vi "splitt argument.vi"(1 "formula":string) -> (0 "Array":string[](array[string]))   [LabVIEW 2011]
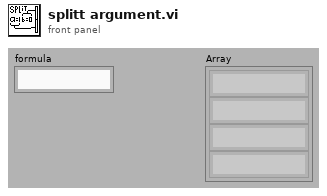
[diagram p1: front panel]
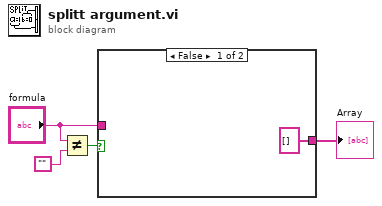
[diagram p0: block diagram]
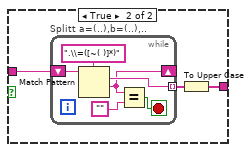
[diagram p2: hidden frame]
diagram:
  n1 = Not Equal?(x="formula", y="") -> (x != y?=w3:bool)
  n2 = case shown="False" w3 {
    tunnel: "formula" -> [_ w8]
    tunnel: [string[] [] w7] -> w4
    frame False {
    }
    frame True {
      n3 = while "Splitt a=(..),b=(..),.." {
        shift-right: [w10] -> _
        shift-left: w8 -> [w14]
        tunnel: [w12] -> w6 mode=indexing
        stop <- w9 stop-if-true
        n4 = Match Pattern(string=w14, regular expression=".\\=([~( )]*)") -> (match substring=w12:string, after substring=w10:string)  [unwired: 1 in, 2 out]
        n5 = Equal?(x=w10, y="") -> (x = y?=w9:bool)
      }
      n6 = To Upper Case(1:w6) -> (0:w7:string[])
    }
  }
  "Array" <- w4
